vi "구조공부-1.vi"() -> ()   [LabVIEW 2018]
uses:
  <vilib>/LabVIEW Open Source Project/MQTT TCP Connection/MQTT_TCP/Connection/TCPConnection.lvclass
  C:/Program Files (x86)/National Instruments/LabVIEW 2018/vi.lib/LabVIEW Open Source Project/Connection/Connection/Connection.lvclass
  auto_update_server/Module/Message Queue/Enqueue Message (Single).vi
  <vilib>/LabVIEW Open Source Project/Connection/Connection/Connection.lvclass
  auto_update_server/Module/Message Queue/Message Queue.lvlib
panel:
  out "문자열 2":string
  out "listener error 2":errorcluster
  in  "정지":bool
  out "server session error 2":errorcluster
  out "server connected 2":bool
  out "ccc":bool
  out "bbb":bool
  out "aaa":bool
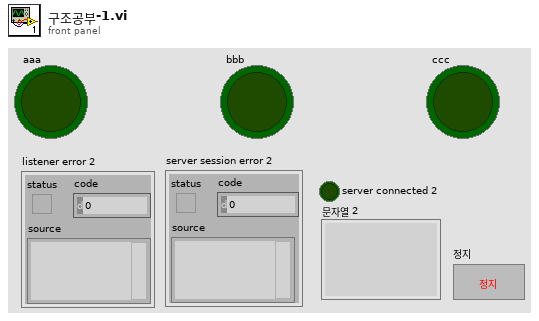
[diagram p1: front panel]
types:
  T1 = typedef "장난감컨트롤.ctl" = enum16{"대기", "연결됨", "연결종료", "종료"}
  T2 = typedef "Message Queue.lvlib/All Message Queues.ctl" = cluster{"UI":refnum<queue>, "Display":refnum<queue>, "Timer":refnum<queue>}
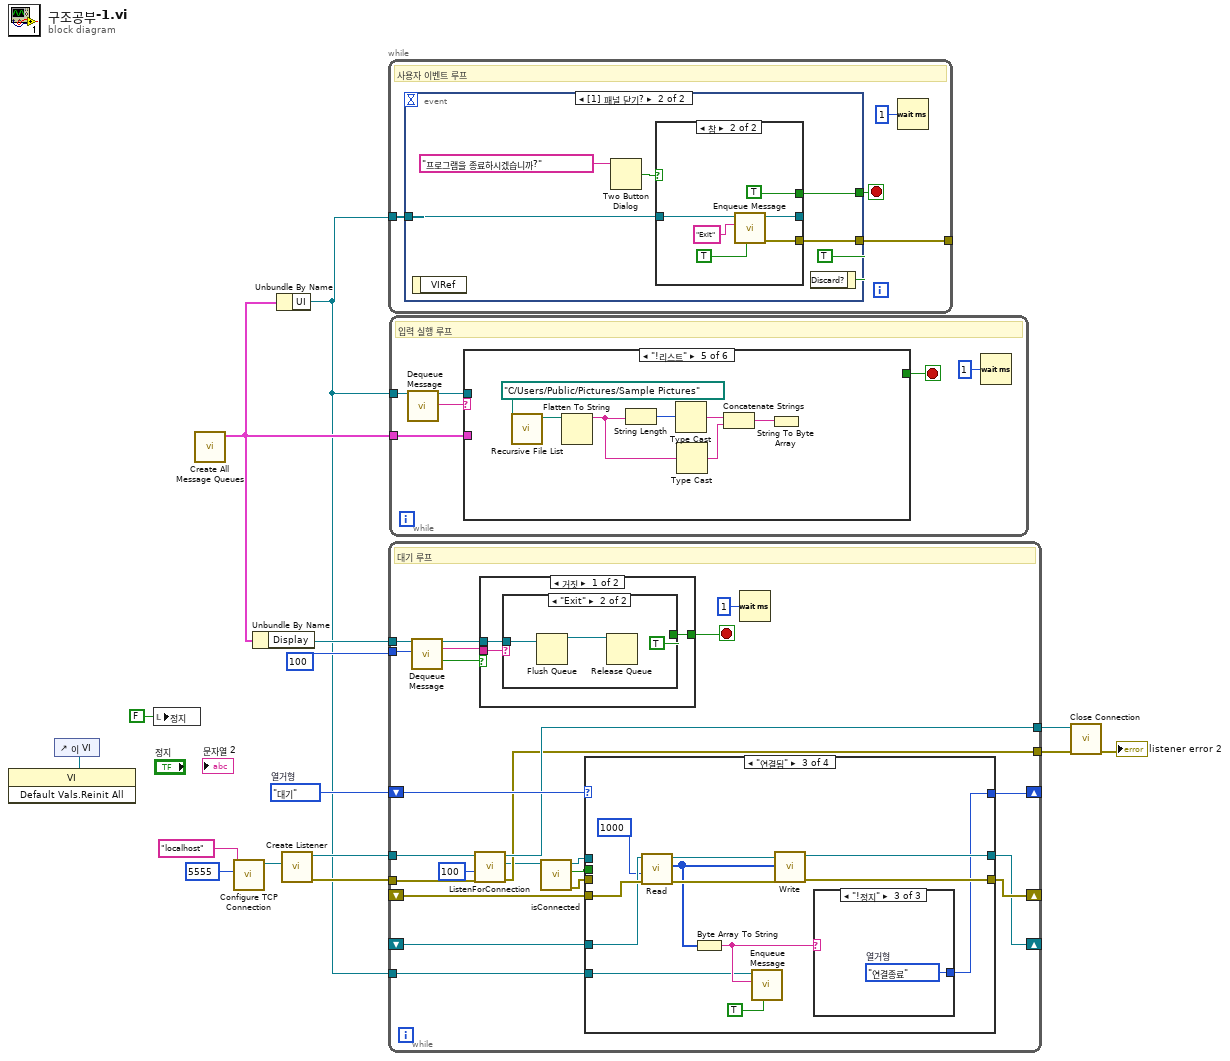
[diagram p0: block diagram]
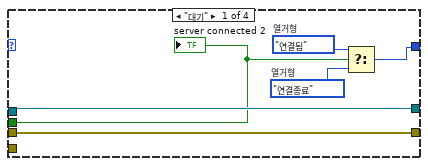
[diagram p4: hidden frame]
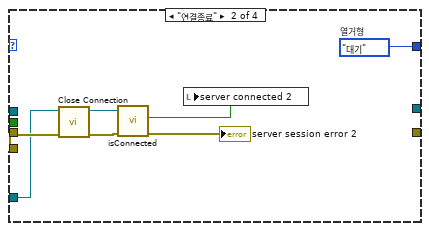
[diagram p5: hidden frame]
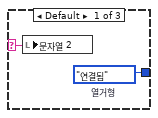
[diagram p6: hidden frame]
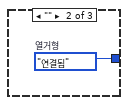
[diagram p7: hidden frame]
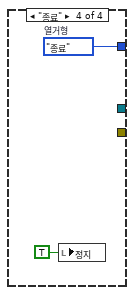
[diagram p8: hidden frame]
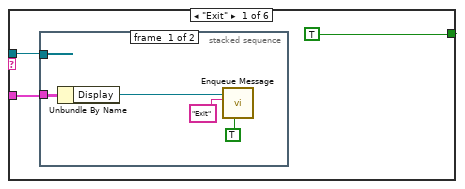
[diagram p9: hidden frame]
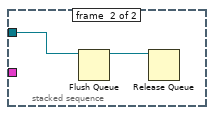
[diagram p10: hidden frame]
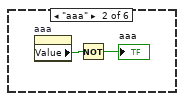
[diagram p11: hidden frame]
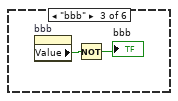
[diagram p12: hidden frame]
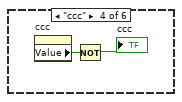
[diagram p13: hidden frame]
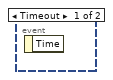
[diagram p15: hidden frame]
diagram:
  w6 = 장난감컨트롤."대기"  # 열거형
  n1 = control-ref of="이 VI"() -> (w11:refnum<vi>)
  n2 = invoke class="VI" method="Default Vals.Reinit All"(reference=w11) -> ()  [unwired: 2 in, 3 out]
  n3 = local write "정지"(FALSE ("정지")) -> ()
  n4 = call "Create All Message Queues.vi"() -> ("Message Queues out"=w15:T2)  [unwired: 10 in, 1 out]
  n5 = call <vilib>:"Configure TCP Connection.vi"("remote port (80)"=u16 5555, "address (localhost)"="localhost") -> ("TCPConnection"=w14:refnum<class "TCPConnection.lvclass">)  [unwired: 8 in, 1 out]
  n6 = Unbundle By Name(w15) -> ("Display"=w2:refnum<queue>)
  n7 = Unbundle By Name(w15) -> ("UI"=w1:refnum<queue>)
  n8 = call <vilib>:"Create Listener.vi"("Connection Configuration"=w14) -> ("error out"=w5:errorcluster, "Listener"=w4:refnum<class "TCPConnection.lvclass">)  [unwired: 9 in]
  n9 = while "While 루프" {
    tunnel: [w19] -> _
    tunnel: w1 -> [w18]
    stop <- w17 stop-if-true
    # "사용자 이벤트 루프"
    n10 = event shown="[1] 패널 닫기?" {
      selector: _ -> [_ _]
      dyn-events: _ -> [_ _]
      timeout: _ -> [_ _]
      tunnel: [_ w22] -> w19
      tunnel: w18 -> [_ w21]
      tunnel: [_ w20] -> w17
      event Timeout {
        n11 = event-data() -> ()  [unwired: 1 in, 1 out]
      }
      event Panel Close? {
        n12 = event-data() -> ()  [unwired: 1 in, 1 out]
        n13 = Two Button Dialog(message="프로그램을 종료하시겠습니까?" ("메시지")) -> (T button?=w23:bool)  [unwired: 2 in]
        n14 = case shown="참" w23 {
          tunnel: [_ w30] -> w22
          tunnel: [_ TRUE] -> w20
          tunnel: w21 -> [w26 w28]
          tunnel: [w26 w27] -> _
          frame False {
          }
          frame True {
            n15 = call-poly "Enqueue Message.vi"("Priority Message? (F)"=TRUE, "Message"="Exit", "Message Queue"=w28) -> ("error out"=w30:errorcluster, "dup Message Queue"=w27:refnum<queue>)  [unwired: 7 in]
          }
        }
        n16 = event-data("Discard?"=TRUE ("버림?")) -> ()  [unwired: 1 in, 1 out]
      }
    }
    n17 = Wait (ms)(milliseconds to wait=u32 1 ("대기 시간 (ms)")) -> ()  [unwired: 1 out]
  }
  n18 = while {
    tunnel: [w53] -> w8
    tunnel: [w51] -> w7
    shift-right: [w54] -> _
    shift-left: w6 -> [w55]
    tunnel: w5 -> [w52]
    shift-right: [w50] -> _
    shift-left: _ -> [w49]
    tunnel: w4 -> [w44]
    shift-right: [w43] -> _
    shift-left: _ -> [w42]
    tunnel: w1 -> [w41]
    tunnel: 100 ("타임아웃(ms) (-1)") -> [w35]
    tunnel: w2 -> [w34]
    stop <- w36 stop-if-true
    # "대기 루프"
    n19 = call "Dequeue Message.vi"("Message Queue"=w34, "타임아웃(ms) (-1)"=w35) -> ("dup Message Queue"=w38:refnum<queue>, "Message"=w39:string, "타임아웃?"=w40:bool)  [unwired: 9 in, 2 out]
    n20 = call <vilib>:"ListenForConnection.vi"("error in (no error)"=w52, "timeout (2000 ms)"=100, "Listener"=w44) -> ("error out"=w51:errorcluster, "Connection"=w48:refnum<class "Connection.lvclass">, "Listener out"=w53:refnum<class "TCPConnection.lvclass">)  [unwired: 5 in, 1 out]
    n21 = case shown="거짓" w40 {
      tunnel: w39 -> [w58 _]
      tunnel: w38 -> [w57 _]
      tunnel: [w56 _] -> w36
      frame False {
        n22 = case shown="\"Exit\"" w58 {
          tunnel: w57 -> [_ w60]
          tunnel: [_ TRUE] -> w56
          frame Default {
          }
          frame "Exit" {
            n23 = Flush Queue(queue=w60) -> (queue out=w61:refnum<queue>)  [unwired: 1 in, 2 out]
            n24 = Release Queue(queue=w61) -> ()  [unwired: 2 in, 3 out]
          }
        }
      }
      frame True {
      }
    }
    n25 = call <vilib>:"isConnected.vi"("Connection in"=w48) -> ("error out"=w47:errorcluster, "connected"=w46:bool, "Connection out"=w33:refnum<class "Connection.lvclass">)  [unwired: 8 in]
    n26 = case shown="\"연결됨\"" w55 {
      tunnel: [w67 w70 w78 w92] -> w54
      tunnel: [w64 _ w81 _] -> w43
      tunnel: [w62 _ w84 _] -> w50
      tunnel: w49 -> [_ w69 w86 _]
      tunnel: w33 -> [w64 _ _ _]
      tunnel: w47 -> [w62 _ _ _]
      tunnel: w46 -> [w63 _ _ _]
      tunnel: w42 -> [_ w68 w83 _]
      tunnel: w41 -> [_ _ w75 _]
      frame "대기" {
        w65 = 장난감컨트롤."연결종료"  # 열거형
        w66 = 장난감컨트롤."연결됨"  # 열거형
        n27 = Select(t=w66, s=w63, f=w65) -> (s? t:f=w67:T1)
        "server connected 2" <- w63
      }
      frame "연결종료" {
        w70 = 장난감컨트롤."대기"  # 열거형
        n28 = call <vilib>:"Close Connection.vi"("error in (no error)"=w69, "Connection in"=w68) -> ("error out"=w71:errorcluster, "No Connection"=w73:refnum<class "Connection.lvclass">)  [unwired: 8 in]
        n29 = call <vilib>:"isConnected.vi"("error in (no error)"=w71, "Connection in"=w73) -> ("error out"=→"server session error 2":errorcluster, "connected"=w74:bool)  [unwired: 7 in, 1 out]
        n30 = local write "server connected 2"(w74) -> ()
      }
      frame "연결됨" {
        n31 = call <vilib>:"Read.vi"("error in (no error)"=w86, "timeout (2000 ms)"=1000, "TCPConnection in"=w83) -> ("error out"=w85:errorcluster, "Bytes"=w79:u8[], "TCPConnection out"=w82:refnum<class "Connection.lvclass">)  [unwired: 4 in, 2 out]
        n32 = Byte Array To String(unsigned byte array=w79) -> (string=w76:string)
        n33 = call-poly "Enqueue Message.vi"("Priority Message? (F)"=TRUE, "Message"=w76, "Message Queue"=w75) -> ()  [unwired: 7 in, 2 out]
        n34 = call <vilib>:"Write.vi"("error in (no error)"=w85, "Bytes"=w79, "Connection in"=w82) -> ("error out"=w84:errorcluster, "Connection"=w81:refnum<class "Connection.lvclass">)  [unwired: 7 in]
        n35 = case shown="\"!정지\"" w76 {
          selector: w76 -> [w88 _ _]
          tunnel: [w87 w89 w90] -> w78
          frame Default {
            w87 = 장난감컨트롤."연결됨"  # 열거형
            n36 = local write "문자열 2"(w88) -> ()
          }
          frame "" {
            w89 = 장난감컨트롤."연결됨"  # 열거형
          }
          frame "!정지" {
            w90 = 장난감컨트롤."연결종료"  # 열거형
          }
        }
      }
      frame "종료" {
        w92 = 장난감컨트롤."종료"  # 열거형
        n37 = local write "정지"(TRUE ("정지")) -> ()
      }
    }
    n38 = Wait (ms)(milliseconds to wait=u32 1 ("대기 시간 (ms)")) -> ()  [unwired: 1 out]
  }
  n39 = while {
    tunnel: w1 -> [w98]
    tunnel: w15 -> [w96]
    stop <- w94 stop-if-true
    # "입력 실행 루프"
    n40 = call "Dequeue Message.vi"("Message Queue"=w98) -> ("dup Message Queue"=w95:refnum<queue>, "Message"=w97:string)  [unwired: 10 in, 3 out]
    n41 = case shown="\"!리스트\"" w97 {
      tunnel: w96 -> [w101 _ _ _ _ _]
      tunnel: w95 -> [w100 _ _ _ _ _]
      tunnel: [TRUE _ _ _ _ _] -> w94
      frame "Exit" {
        n42 = stacked-sequence {
          tunnel: w101 -> [w105 _]
          tunnel: w100 -> [_ w107]
          frame #0 {
            n43 = Unbundle By Name(w105) -> ("Display"=w104:refnum<queue>)
            n44 = call-poly "Enqueue Message.vi"("Priority Message? (F)"=TRUE, "Message"="Exit", "Message Queue"=w104) -> ()  [unwired: 7 in, 2 out]
          }
          frame #1 {
            n45 = Flush Queue(queue=w107) -> (queue out=w106:refnum<queue>)  [unwired: 1 in, 2 out]
            n46 = Release Queue(queue=w106) -> ()  [unwired: 2 in, 3 out]
          }
        }
      }
      frame "aaa" {
        n47 = property on="aaa" class="Bool (엄격한)"() -> ("Value"=w109:bool)  [unwired: 2 in, 2 out]
        n48 = Not(x=w109) -> (.not. x?=→"aaa":bool)
      }
      frame "bbb" {
        n49 = property on="bbb" class="Bool (엄격한)"() -> ("Value"=w111:bool)  [unwired: 2 in, 2 out]
        n50 = Not(x=w111) -> (.not. x?=→"bbb":bool)
      }
      frame "ccc" {
        n51 = property on="ccc" class="Bool (엄격한)"() -> ("Value"=w113:bool)  [unwired: 2 in, 2 out]
        n52 = Not(x=w113) -> (.not. x?=→"ccc":bool)
      }
      frame "!리스트" {
        n53 = call <vilib>:"Recursive File List.vi"("Folder Path"=path "C:/Users/Public/Pictures/Sample Pictures") -> ("dup Folder Path"=w120:path)  [unwired: 6 in, 4 out]
        n54 = Flatten To String(anything=w120) -> (data string=w117:string)  [unwired: 3 in, 2 out]
        n55 = String Length(string=w117) -> (length=w119:i32)
        n56 = Type Cast(x=w119) -> (*(type *) &x=w118:string)  [unwired: 1 in]
        n57 = Type Cast(x=w117) -> (*(type *) &x=w116:string)  [unwired: 1 in]
        n58 = Concatenate Strings(w118, w116) -> (w115:string)
        n59 = String To Byte Array(string=w115) -> ()  [unwired: 1 out]
      }
      frame Default {
      }
    }
    n60 = Wait (ms)(milliseconds to wait=u32 1 ("대기 시간 (ms)")) -> ()  [unwired: 1 out]
  }
  n61 = call <vilib>:"Close Connection.vi"("error in (no error)"=w7, "Connection in"=w8) -> ("error out"=→"listener error 2":errorcluster)  [unwired: 8 in, 1 out]
